vi "Initialize.vi"(8 "error in (no error)":errorcluster, 10 "Communication variables":T1={"FWCS IP"="200.131.64.49", "ACS IP"="200.131.64.49", "Channel ID"=1} {"Channel ID" min=1}, 11 "SPARC4_GUI in":refnum<class "S4GEI.lvclass">) -> (0 "error out":errorcluster, 3 "SPARC4_GUI out":refnum<class "S4GEI.lvclass">)   [LabVIEW 2018, in "S4GEI.lvclass"]
uses:
  S4GEI.lvclass
  S4GEI.lvclass/S4GEI.ctl
  Channel GUI/Channel.lvclass/Channel.ctl
  Channel GUI/Channel.lvclass
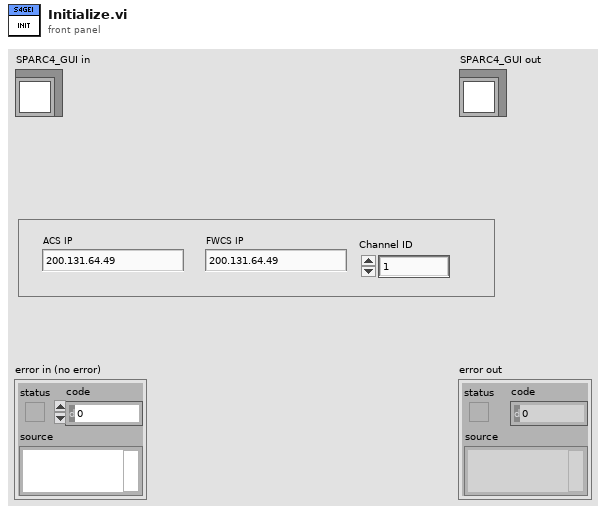
[diagram p1: front panel]
types:
  T1 = cluster{"FWCS IP":string, "ACS IP":string, "Channel ID":u16}
  T2 = cluster{"OBJECT":string, "OBSERVER":string, "CTRLINTE":string, "PROJID":string, "SYNCMODE":string, "INSTMODE":string, "FILTER":string, "OBSTYPE":string, "GUIVRSN":string, "COMMENT":string, "broker":string, "timestamp":string, "CHANNEL 1":bool, "CHANNEL 2":bool, "CHANNEL 3":bool, "CHANNEL 4":bool, "TCSMODE":bool}
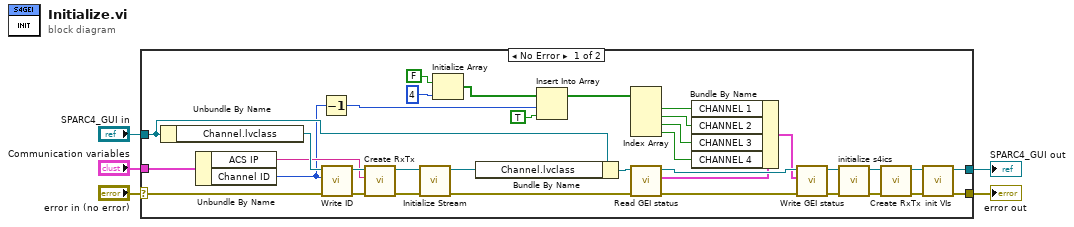
[diagram p0: block diagram]
diagram:
  n1 = case shown="No Error" "error in (no error)" {
    selector: "error in (no error)" -> [w38 w42]
    tunnel: [w6 w42] -> w4
    tunnel: [w7 w41] -> w2
    tunnel: "SPARC4_GUI in" -> [w40 w41]
    tunnel: "Communication variables" -> [w31 _]
    frame No Error {
      n2 = Unbundle By Name(w40) -> ("Channel.lvclass"=w39:refnum<class "Channel.lvclass">)
      n3 = Unbundle By Name(w31) -> ("ACS IP"=w32:string, "Channel ID"=w13:u16)
      n4 = Decrement(x=w13) -> (x-1=w14:u16)
      n5 = call "Write ID.vi"("error in (no error)"=w38, "ID"=w13, "Channel GUI in"=w39) -> ("error out"=w33:errorcluster, "Channel GUI out"=w36:refnum<class "Channel.lvclass">)  [unwired: 7 in]
      n6 = call "Create RxTx.vi"("error in (no error)"=w33, "Remote IP"=w32, "Channel GUI in"=w36) -> ("error out"=w34:errorcluster, "Channel GUI out"=w35:refnum<class "Channel.lvclass">)  [unwired: 7 in]
      n7 = call "Initialize Stream.vi"("error in (no error)"=w34, "Channel GUI in"=w35) -> ("error out"=w22:errorcluster, "Channel GUI out"=w37:refnum<class "Channel.lvclass">)  [unwired: 8 in]
      n8 = Initialize Array(FALSE, 4 ("dimension size")) -> (w16:bool[])
      n9 = Bundle By Name(cluster=w40, "Channel.lvclass"=w37) -> (w23:refnum<class "S4GEI.lvclass">)
      n10 = Insert Into Array(array=w16, index=w14, new element=TRUE) -> (w12:bool[])
      n11 = Index Array(array=w12) -> (element #1=w11:bool, element #2=w10:bool, element #3=w9:bool, element #4=w8:bool)  [unwired: 4 in]
      n12 = call-dynamic "Read GEI status.vi"("error in (no error)"=w22, "S4GEI in"=w23) -> ("error out"=w21:errorcluster, "GEI status"=w20:T2, "S4GEI out"=w24:refnum<class "S4GEI.lvclass">)  [unwired: 7 in]
      n13 = Bundle By Name(cluster=w20, "CHANNEL 1"=w11, "CHANNEL 2"=w10, "CHANNEL 3"=w9, "CHANNEL 4"=w8) -> (w19:T2)
      n14 = call-dynamic "Write GEI status.vi"("error in (no error)"=w21, "GEI status"=w19, "S4GEI in"=w24) -> ("error out"=w26:errorcluster, "S4GEI out"=w25:refnum<class "S4GEI.lvclass">)  [unwired: 7 in]
      n15 = call "initialize s4ics.vi"("error in (no error)"=w26, "S4GEI in"=w25) -> ("error out"=w27:errorcluster, "S4GEI out"=w28:refnum<class "S4GEI.lvclass">)  [unwired: 8 in]
      n16 = call "Create RxTx.vi"("error in (no error)"=w27, "S4GEI in"=w28) -> ("error out"=w29:errorcluster, "S4GEI out"=w30:refnum<class "S4GEI.lvclass">)  [unwired: 8 in]
      n17 = call "init VIs.vi"("error in (no error)"=w29, "S4GEI in"=w30) -> ("error out"=w6:errorcluster, "S4GEI out"=w7:refnum<class "S4GEI.lvclass">)  [unwired: 8 in]
    }
    frame Error {
    }
  }
  "error out" <- w4
  "SPARC4_GUI out" <- w2
